vi "Check_For_Illegal_Conpane_Types.vi"(8 "error in (no error)":errorcluster, 11 "VI in":refnum<vi>) -> (0 "error out":errorcluster, 2 "Error Message":string, 3 "VI out":refnum<vi>)   [LabVIEW 2020, in "AB_DLL.lvclass"]
uses:
  <vilib>/AppBuilder/AB_Classes/DLL/AB_DLL.lvclass
  <resource>/Framework/Providers/Common/provcom_StringGlobals.vi
  <vilib>/Utility/Data Type/NI_Data Type.lvlib
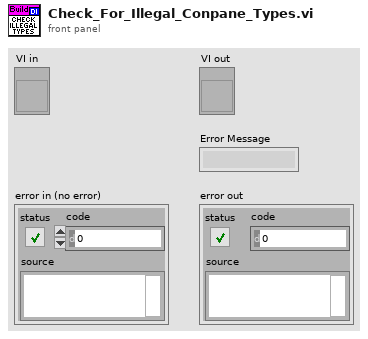
[diagram p1: front panel]
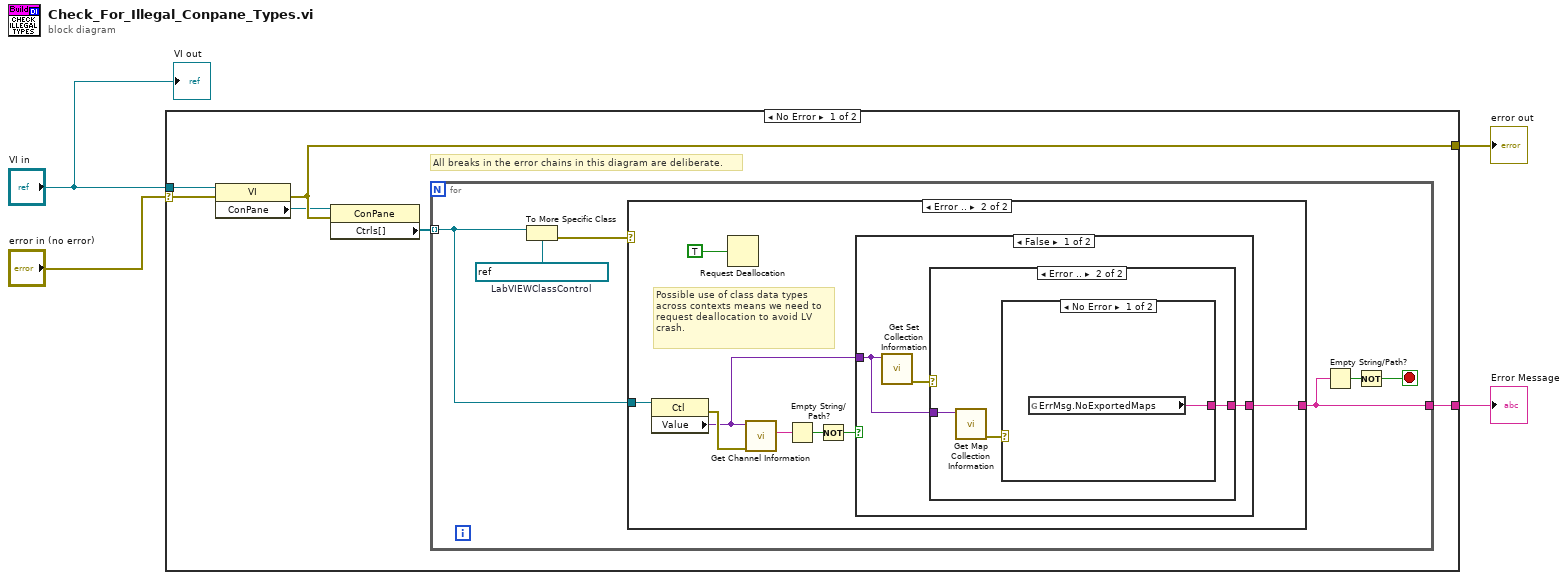
[diagram p0: block diagram]
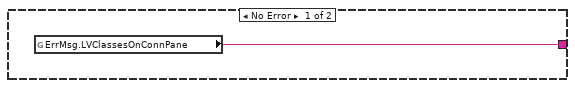
[diagram p2: hidden frame]
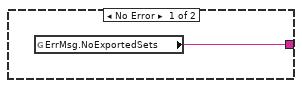
[diagram p3: hidden frame]
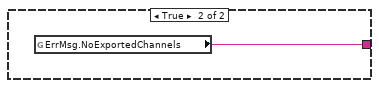
[diagram p5: hidden frame]
diagram:
  n1 = case shown="No Error" "error in (no error)" {
    selector: "error in (no error)" -> [w8 w35]
    tunnel: "VI in" -> [w9 _]
    tunnel: [w10 w35] -> w3
    tunnel: [w5 _] -> w2
    frame No Error {
      # "All breaks in the error chains in this diagram are deliberate."
      n2 = property class="VI"(reference=w9, error in=w8) -> (error out=w10:errorcluster, "ConPane"=w7:refnum<vi>)  [unwired: 1 out]
      n3 = property class="ConPane"(reference=w7, error in=w10) -> ("Ctrls[]"=w6:refnum<vi>[])  [unwired: 2 out]
      n4 = for {
        tunnel: w6 -> [w14] mode=indexing
        tunnel: [w12] -> w5
        stop <- w11 stop-if-true
        w16 = refnum<vi> refnum  # LabVIEWClassControl
        n5 = To More Specific Class(target class=w16, reference=w14) -> (error out=w15:errorcluster)  [unwired: 1 in, 1 out]
        n6 = case shown="Error .." w15 {
          tunnel: [w17 w25] -> w12
          tunnel: w14 -> [_ w21]
          frame No Error {
            n7 = global read "provcom_StringGlobals.vi" "ErrMsg.LVClassesOnConnPane"() -> (w17:string)
          }
          frame Error {
            # "Possible use of class data types across contexts means we need to request deallocation to avoid LV crash."
            n8 = property class="Ctl"(reference=w21) -> (error out=w24:errorcluster, "Value"=w19:variant)  [unwired: 1 in, 1 out]
            n9 = Request Deallocation(TRUE ("flag")) -> ()
            n10 = call <vilib>:"Get Channel Information.vi"("error in (no error)"=w24, "variant"=w19) -> ("template name"=w23:string)  [unwired: 5 in, 4 out]
            n11 = Empty String/Path?(string/path=w23) -> (empty?=w22:bool)
            n12 = Not(x=w22) -> (.not. x?=w20:bool)
            n13 = case shown="False" w20 {
              tunnel: [w27 w34] -> w25
              tunnel: w19 -> [w26 _]
              frame False {
                n14 = call <vilib>:"Get Set Collection Information.vi"("variant"=w26) -> ("error out"=w28:errorcluster)  [unwired: 9 in, 1 out]
                n15 = case shown="Error .." w28 {
                  tunnel: [w29 w30] -> w27
                  tunnel: w26 -> [_ w32]
                  frame No Error {
                    n16 = global read "provcom_StringGlobals.vi" "ErrMsg.NoExportedSets"() -> (w29:string)
                  }
                  frame Error {
                    n17 = call <vilib>:"Get Map Collection Information.vi"("variant"=w32) -> ("error out"=w31:errorcluster)  [unwired: 8 in, 2 out]
                    n18 = case shown="No Error" w31 {
                      tunnel: [w33 _] -> w30
                      frame No Error {
                        n19 = global read "provcom_StringGlobals.vi" "ErrMsg.NoExportedMaps"() -> (w33:string)
                      }
                      frame Error {
                      }
                    }
                  }
                }
              }
              frame True {
                n20 = global read "provcom_StringGlobals.vi" "ErrMsg.NoExportedChannels"() -> (w34:string)
              }
            }
          }
        }
        n21 = Empty String/Path?(string/path=w12) -> (empty?=w13:bool)
        n22 = Not(x=w13) -> (.not. x?=w11:bool)
      }
    }
    frame Error {
    }
  }
  "error out" <- w3
  "Error Message" <- w2
  "VI out" <- "VI in"
